vi "gds_usrp_rx.vi"() -> ()   [LabVIEW 2012]
uses:
  <instrlib>/niUSRP/niUSRP Fetch Rx Data (CDB Cluster).vi
  <vilib>/addons/Modulation/niDMT.lvlib
panel:
  in  "autoscale":bool
  out "Constellation Graph":T1(graph)
  in  "stop":bool
  out "Key Bit Sequence":i8[](array[numeric])
  in  "active antenna":string="RX2"
  out "coerced gain":dbl format="%#_6f"
  out "coerced carrier frequency":dbl=100000.0 format="%#_6p"
  out "coerced IQ rate":dbl=100000.0 format="%#_6p"
  in  "gain":dbl=20.0 format="%#_6f"
  in  "carrier frequency":dbl=433000000.0 format="%#_6p"
  out "Recoverd Bit Sequence":i8[](array[numeric])=[1, 0, 1, 0, 0, 0, 1, 1, 0] caption="Recovered Bit Sequence"
  out "Measurements":T2 caption="measurements" {"FSK error (Hz)" format="%.2f"; "deviation error (Hz)" format="%.2f"; "frequency drift (Hz)" format="%.2f"; "frequency offset (Hz)" format="%.2f"}
  out "BER":dbl
  in  "Modulation Parameters":T3={"RX Parameters"={"Sampling Rate"=1000000.0, "RX Oversample Factor"=2}, "Shared Parameters"={"Packet Length"=500, "Preamble Length"=20, "modulation type"=enum."OOK", "FSK deviation (Hz)"=625.0, "Filter Parameters"={"modulation type"=enum."ASK", "pulse shaping filter (none)"=enum."none", "filter length (symbols)"=8, "filter parameter"=0.5}}}
  in  "device names":refnum<k15>="192.168.10.26"
  out "error out":errorcluster
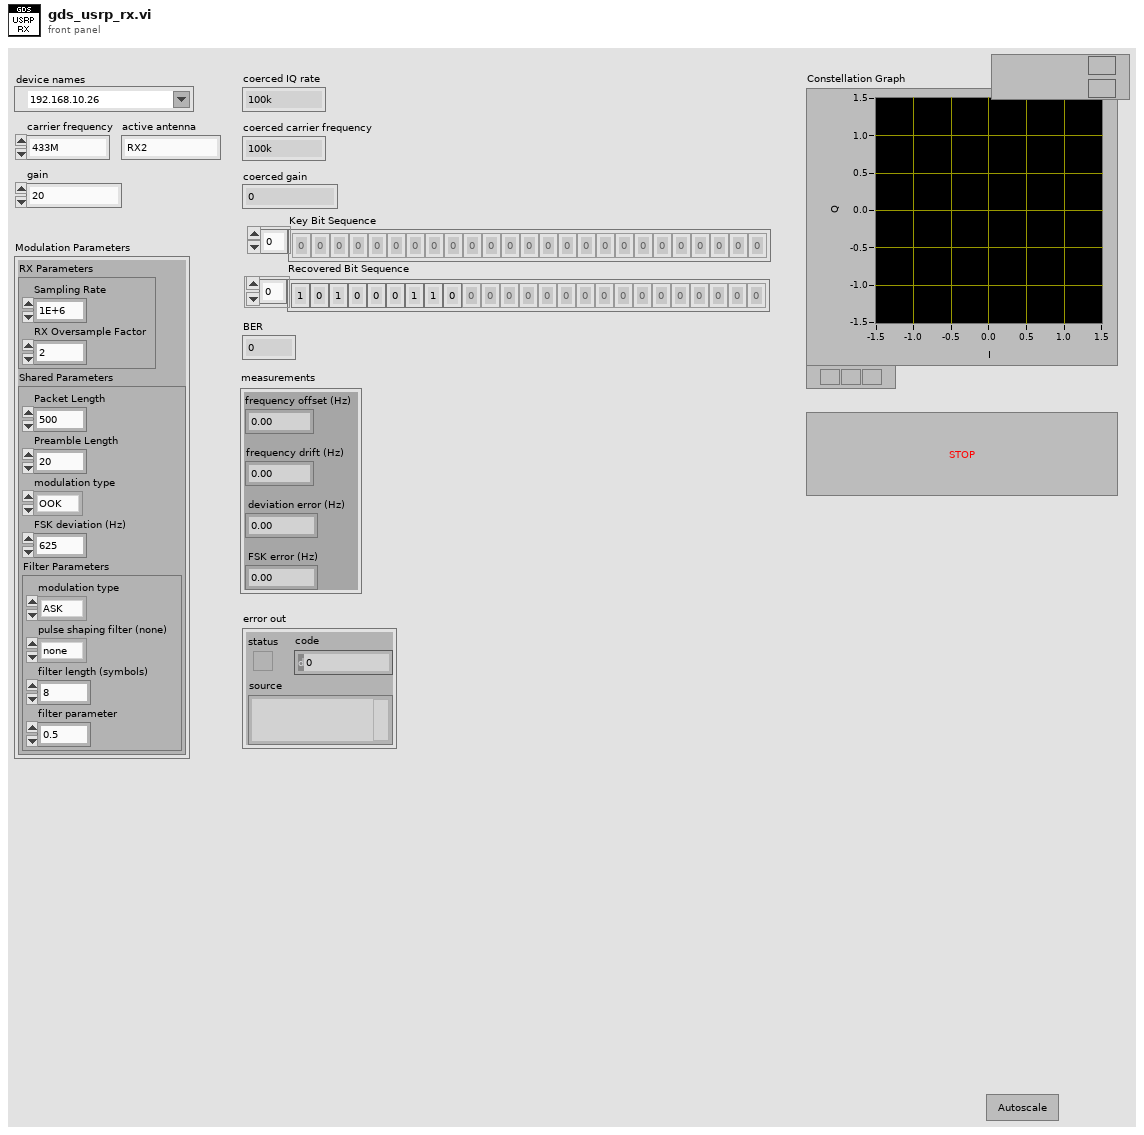
[diagram p1: front panel]
types:
  T1 = cluster{"Decimated Array":dbl[], "Decimated Array":dbl[]}[]
  T2 = cluster{"frequency offset (Hz)":dbl, "frequency drift (Hz)":dbl, "deviation error (Hz)":dbl, "FSK error (Hz)":dbl}
  T3 = cluster{"RX Parameters":cluster{"Sampling Rate":dbl, "RX Oversample Factor":i32}, "Shared Parameters":cluster{"Packet Length":i32, "Preamble Length":i32, "modulation type":enum16{"OOK", "FSK", "PSK", "QAM", "MSK", "PAM", "ASK", "CPM"}, "FSK deviation (Hz)":dbl, "Filter Parameters":cluster{"modulation type":enum16{"FSK", "PSK", "QAM", "MSK", "PAM", "ASK", "CPM"}, "pulse shaping filter (none)":enum16{"none", "Raised Cosine", "Root Raised Cos", "Gaussian"}, "filter length (symbols)":i32, "filter parameter":dbl}}}
  T4 = typedef "niAMT.lvlib/Complex Data Waveform.ctl" = cluster{"t0":dbl, "dt":dbl, "Y":cdb[]}
  T5 = cluster{"constellation":dbl[], "oversampled data":dbl[]}[]
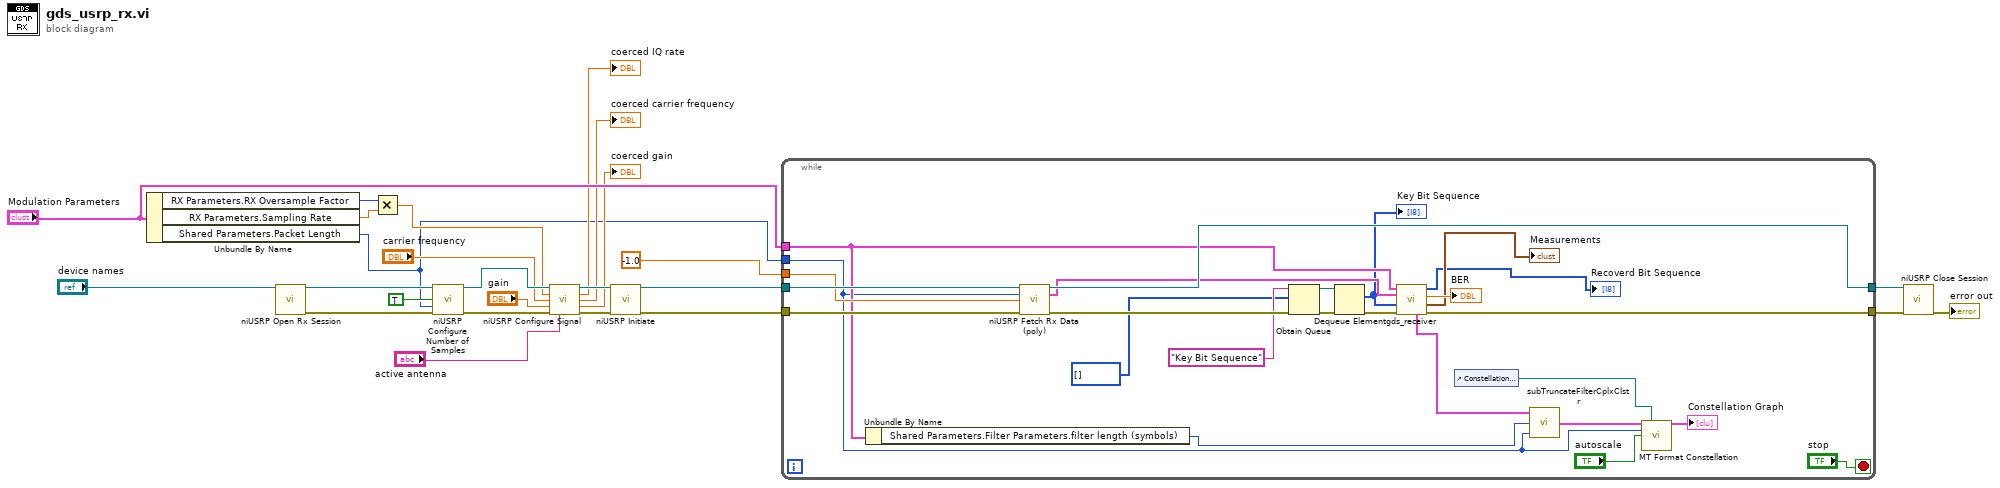
[diagram p0: block diagram]
diagram:
  n1 = Unbundle By Name("Modulation Parameters") -> ("RX Parameters.RX Oversample Factor"=w13:i32, "RX Parameters.Sampling Rate"=w12:dbl, "Shared Parameters.Packet Length"=w2:i32)
  n2 = call <instrlib>:"niUSRP Open Rx Session.vi"("device names"="device names") -> ("session handle out"=w24:refnum<k15>, "error out"=w25:errorcluster)  [unwired: 13 in]
  n3 = Multiply(x=w13, y=w12) -> (x*y=w11:dbl)
  n4 = call <instrlib>:"niUSRP Configure Number of Samples.vi"("session handle"=w24, "number of samples is finite"=TRUE, "number of samples"=w2, "error in (no error)"=w25) -> ("session handle out"=w23:refnum<k15>, "error out"=w22:errorcluster)  [unwired: 10 in]
  n5 = call <instrlib>:"niUSRP Configure Signal.vi"("session handle"=w23, "IQ rate"=w11, "carrier frequency"="carrier frequency", "gain"="gain", "error in (no error)"=w22, "active antenna"="active antenna") -> ("session handle out"=w21:refnum<k15>, "coerced IQ rate"=→"coerced IQ rate":dbl, "coerced carrier frequency"=→"coerced carrier frequency":dbl, "coerced gain"=→"coerced gain":dbl, "error out"=w20:errorcluster)  [unwired: 5 in]
  n6 = call <instrlib>:"niUSRP Initiate.vi"("session handle"=w21, "error in (no error)"=w20) -> ("session handle out"=w3:refnum<k15>, "error out"=w1:errorcluster)  [unwired: 12 in]
  n7 = while {
    tunnel: w3 -> [w50]
    tunnel: w1 -> [w49]
    tunnel: [w48] -> w19
    tunnel: [w47] -> w18
    tunnel: "Modulation Parameters" -> [w32]
    tunnel: w2 -> [w30]
    tunnel: -1.0 ("timeout") -> [w38]
    stop <- "stop" stop-if-true
    n8 = Unbundle By Name(w32) -> ("Shared Parameters.Filter Parameters.filter length (symbols)"=w31:i32)
    n9 = call-poly <instrlib>:"niUSRP Fetch Rx Data (poly).vi"("session handle"=w50, "number of samples"=w30, "timeout"=w38, "error in (no error)"=w49) -> ("session handle out"=w48:refnum<k15>, "data"=w29:cluster{"t0":dbl, "dt":dbl, "Y":cdb[]}, "error out"=w44:errorcluster)  [unwired: 8 in, 1 out]
    n10 = Obtain Queue(name (unnamed)="Key Bit Sequence", element data type=i8[] [], error in (no error)=w44) -> (queue out=w46:refnum<queue>, error out=w45:errorcluster)  [unwired: 2 in, 1 out]
    n11 = Dequeue Element(queue=w46, error in (no error)=w45) -> (element=w27:i8[], error out=w43:errorcluster)  [unwired: 1 in, 2 out]
    "Key Bit Sequence" <- w27
    n12 = call "gds_receiver.vi"("error in (no error)"=w43, "Received Bit Sequence"=w27, "Received Signal"=w29, "Modulation Parameters"=w32) -> ("error out"=w47:errorcluster, "Measurements"=→"Measurements":T2, "BER"=→"BER":dbl, "Key Bit Sequence"=→"Recoverd Bit Sequence":i8[], "recovered complex waveform"=w33:T4)  [unwired: 3 in]
    n13 = control-ref of="Constellation Graph"() -> (w35:refnum<vi>)
    n14 = call "subTruncateFilterCplxClstr.vi"("samples per symbol (16)"=w30, "filter length (symbols)"=w31, "waveform to truncate"=w33) -> ("truncated waveform"=w37:T4)
    n15 = call <vilib>:"MT Format Constellation.vi"("waveform"=w37, "constellation reference"=w35, "samples per symbol"=w30, "autoscale"="autoscale") -> ("constellation graph"=→"Constellation Graph":T5)  [unwired: 10 in, 1 out]
  }
  n16 = call <instrlib>:"niUSRP Close Session.vi"("session handle"=w19, "error in (no error)"=w18) -> ("error out"=→"error out":errorcluster)  [unwired: 13 in]
